vi "PN TYPE.vi"(8 "errin":errorcluster, 10 "Variante":string, 11 "PN":string) -> (0 "error out":errorcluster, 1 "recordset data":variant[][](array[variant]), 2 "chaîne concaténée":string, 3 "Data out":T1)   [LabVIEW 2020]
uses:
  VarGLO/Global var.vi
  <vilib>/addons/database/Connection.llb/DB Tools Open Connec (String).vi
  <vilib>/addons/database/Connection.llb/Conn Execute.vi
  <vilib>/addons/database/Recordset.llb/Rec Fetch Recordset Data (R).vi
  <vilib>/addons/database/Recordset.llb/Rec Destroy - Connection.vi
  <vilib>/addons/database/NI_Database_API.lvlib
panel:
  # "84481"
  # "A"
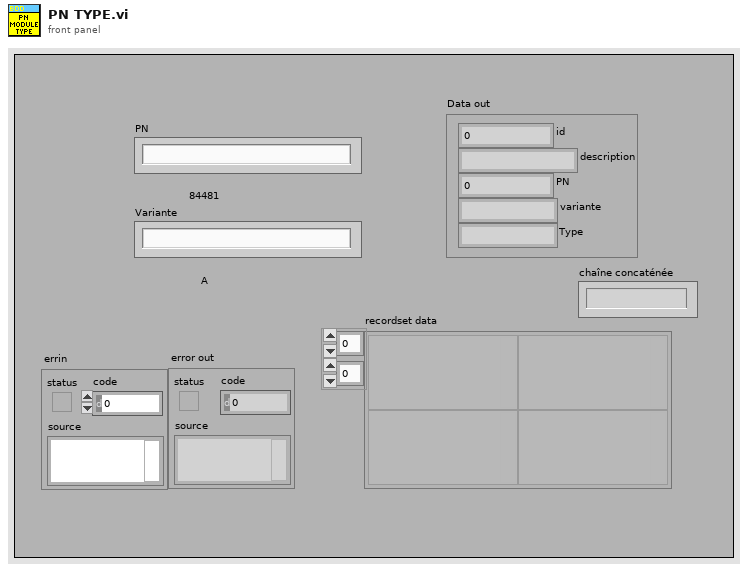
[diagram p1: front panel]
types:
  T1 = cluster{"id":dbl, "description":string, "PN":dbl, "variante":string, "Type":string}
  T2 = typedef "NI_Database_API.lvlib/Conn ObjectReference.ctl" = refnum<k1>
  T3 = typedef "NI_Database_API.lvlib/Rec ObjectReference.ctl" = refnum<k1>
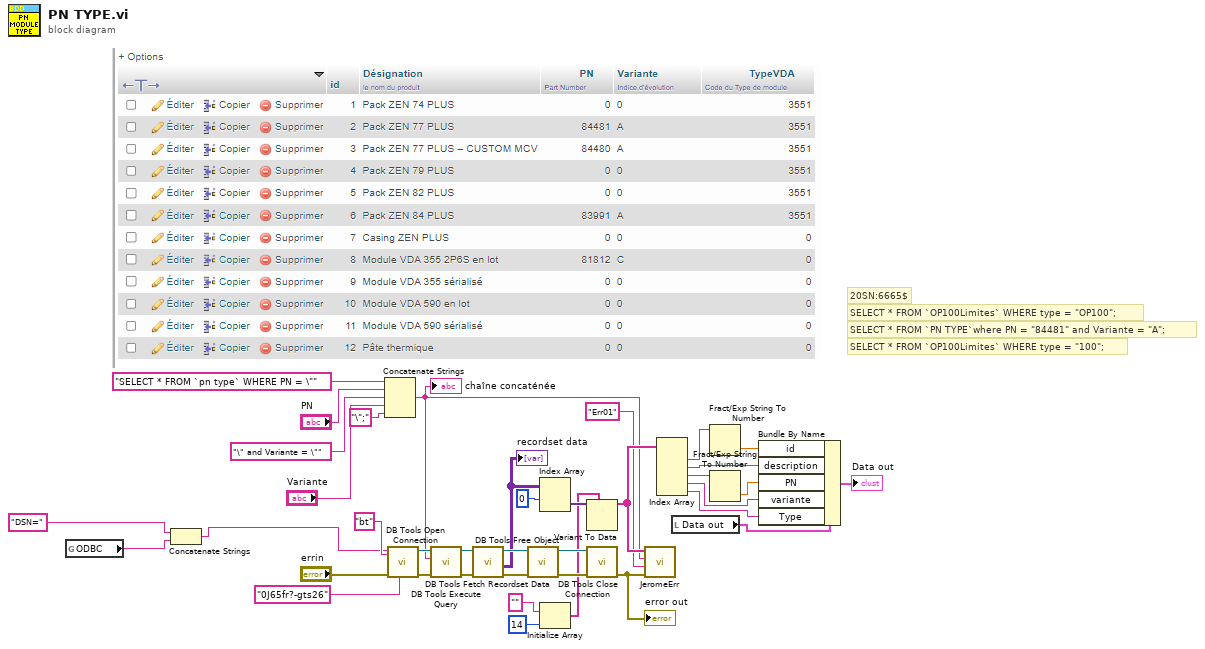
[diagram p0: block diagram]
diagram:
  # "SELECT * FROM `PN TYPE`where PN = \"84481\" and Variante = \"A\";"
  # "SELECT * FROM `OP100Limites` WHERE type = \"OP100\";"
  # "SELECT * FROM `OP100Limites` WHERE type = \"100\";"
  # "20SN:6665$"
  n1 = global read "Global var.vi" "ODBC"() -> (w2:string)
  n2 = Concatenate Strings("DSN=", w2) -> (w1:string)
  n3 = Concatenate Strings("SELECT * FROM `pn type` WHERE PN = \"" ("SQL query"), "PN", "\" and Variante = \"" ("chaîne"), "Variante", "\";" ("chaîne")) -> (w5:string)
  "chaîne concaténée" <- w5
  n4 = call-poly <vilib>:"DB Tools Open Connection.vi"("password"="0J65fr?-gts26", "userID"="bt", "error in (no error)"="errin", "connection information"=w1) -> ("error out"=w38:errorcluster, "connection reference"=w36:T2)  [unwired: 4 in]
  n5 = call-poly <vilib>:"DB Tools Execute Query.vi"("error in (no error)"=w38, "SQL query"=w5, "connection reference"=w36) -> ("error out"=w32:errorcluster, "recordset reference"=w31:T3)  [unwired: 5 in]
  n6 = call-poly <vilib>:"DB Tools Fetch Recordset Data.vi"("error in (no error)"=w32, "recordset reference"=w31) -> ("error out"=w33:errorcluster, "recordset data"=w9:variant[][], "recordset reference out"=w30:T3)  [unwired: 3 in]
  "recordset data" <- w9
  n7 = call-poly <vilib>:"DB Tools Free Object.vi"("error in (no error)"=w33, "recordset reference"=w30) -> ("error out"=w37:errorcluster, "connection reference"=w35:T2)  [unwired: 8 in]
  n8 = Index Array(array=w9, index (row)=0 ("indice (ligne)")) -> (element=w24:variant[])  [unwired: 1 in]
  n9 = Initialize Array("", 14 ("taille de la dimension")) -> (w8:string[])
  n10 = Variant To Data ("Variant en donnée")(type=w8, Variant=w24) -> (data=w6:string[])  [unwired: 1 in, 1 out]
  n11 = call <vilib>:"DB Tools Close Connection.vi"("error in (no error)"=w37, "connection reference"=w35) -> ("error out"=w7:errorcluster)  [unwired: 5 in]
  "error out" <- w7
  n12 = call "JeromeErr.vi"("Errin"=w7, "CodeERR"="Err01", "RequetteSQL"=w5, "RetourSQL"=w6) -> ()  [unwired: 8 in]
  n13 = Index Array(array=w6) -> (element #1=w14:string, element #2=w18:string, element #3=w13:string, element #4=w17:string, element #5=w12:string)  [unwired: 5 in]
  n14 = local read "Data out"() -> (w11:T1)
  n15 = Fract/Exp String To Number(string=w14) -> (number=w16:dbl)  [unwired: 3 in, 1 out]
  n16 = Fract/Exp String To Number(string=w13) -> (number=w15:dbl)  [unwired: 3 in, 1 out]
  n17 = Bundle By Name(cluster=w11, "id"=w16, "description"=w18, "PN"=w15, "variante"=w17, "Type"=w12) -> (→"Data out":T1)
